vi "FGV.vi"(0 "queue in":refnum<queue>, 1 "Action":enum16{"Get", "Set", "Clear"}(ring), 2 "Logger Name":string, 5 "Logger Output in":T1, 7 "Destroy Logger in":bool=TRUE, 9 "Writer ref in":refnum<vi>, 11 "error in (no error)":errorcluster) -> (4 "queue out":refnum<queue>, 6 "Logger Outputs":T1[](array[typedef]), 8 "Destroy Logger out":bool, 10 "Writer ref out":refnum<vi>, 14 "All Named Loggers":variant, 15 "error out":errorcluster)   [LabVIEW 2016, in "Global_logger.lvlib"]
uses:
  Global_logger.lvlib
  Event.ctl
  Levels.ctl
  Logger Output.ctl
  Level Meaning.ctl
  Sorting.ctl
  Logger Type.ctl
  Log Fields.ctl
  <vilib>/Utility/error.llb/Error Cluster From Error Code.vi
  <vilib>/ErrorRing/Error Ring.xnode
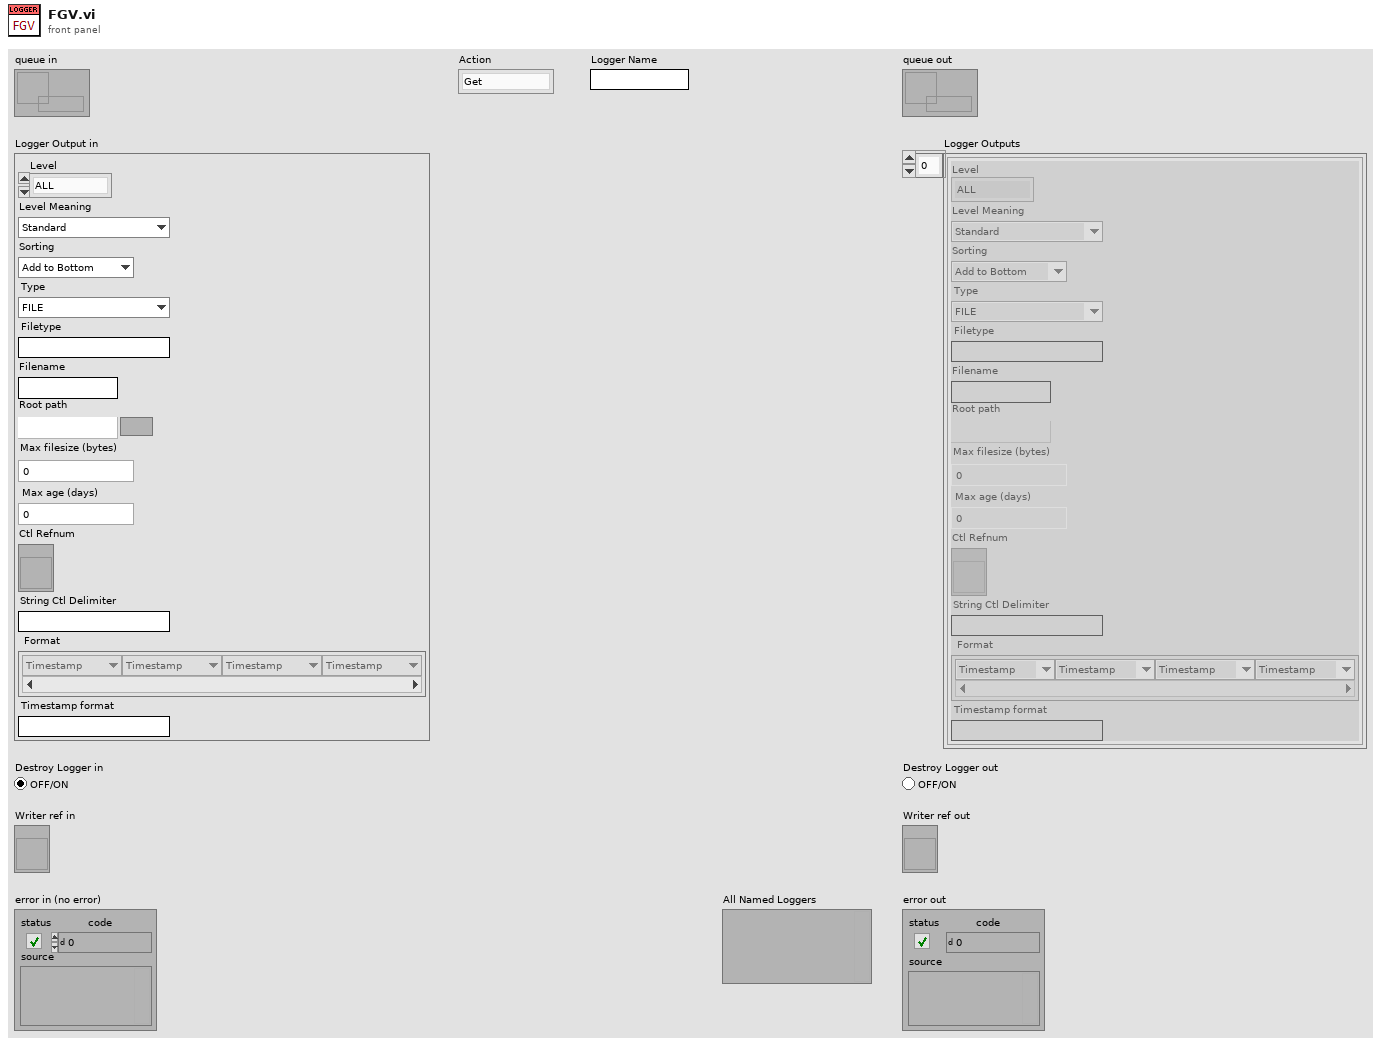
[diagram p1: front panel]
types:
  T1 = typedef "Global_logger.lvlib/Logger Output.ctl" = cluster{"Level":T2, "Level Meaning":T3, "Sorting":T4, "Type":T5, "Filetype":string, "Filename":string, "Root path":path, "Max filesize (bytes)":i32, "Max age (days)":i32, "Ctl Refnum":refnum<vi>, "String Ctl Delimiter":string, "Format":T6[], "Timestamp format":string}
  T2 = typedef "Global_logger.lvlib/Levels.ctl" = enum16{"ALL", "TRACE", "DEBUG", "INFO", "WARN", "ERROR", "FATAL", "OFF"}
  T3 = typedef "Global_logger.lvlib/Level Meaning.ctl" = enum16{"Standard", "Positive", "Exact"}
  T4 = typedef "Global_logger.lvlib/Sorting.ctl" = enum16{"Add to Bottom", "Add to Top"}
  T5 = typedef "Global_logger.lvlib/Logger Type.ctl" = enum16{"FILE", "UI"}
  T6 = typedef "Global_logger.lvlib/Log Fields.ctl" = enum16{"Timestamp", "Level", "Message", "Source VI", "Source App", "Logger Name"}
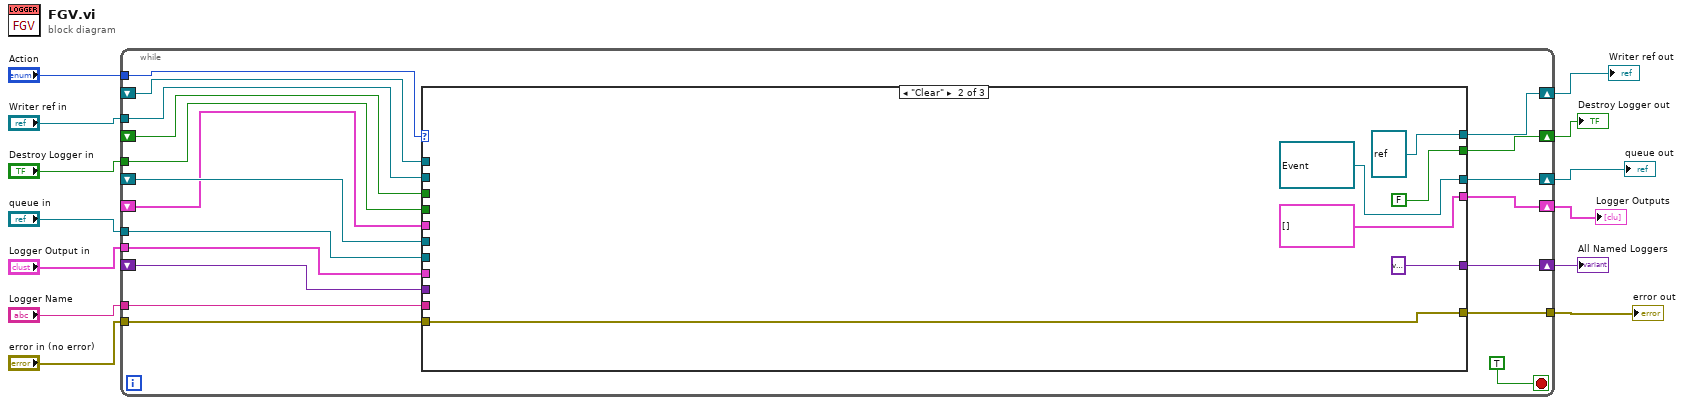
[diagram p0: block diagram]
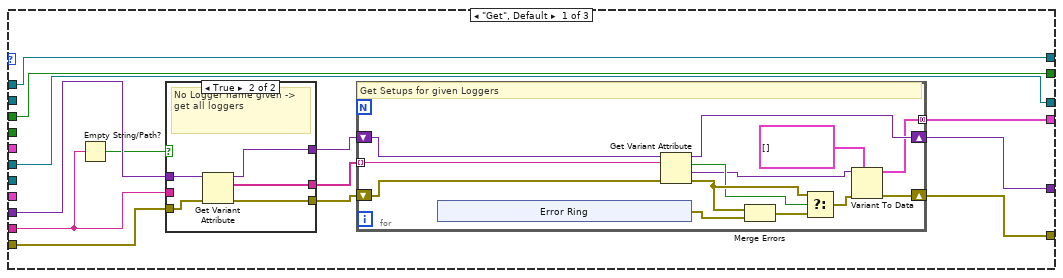
[diagram p2: hidden frame]
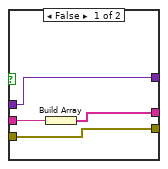
[diagram p3: hidden frame]
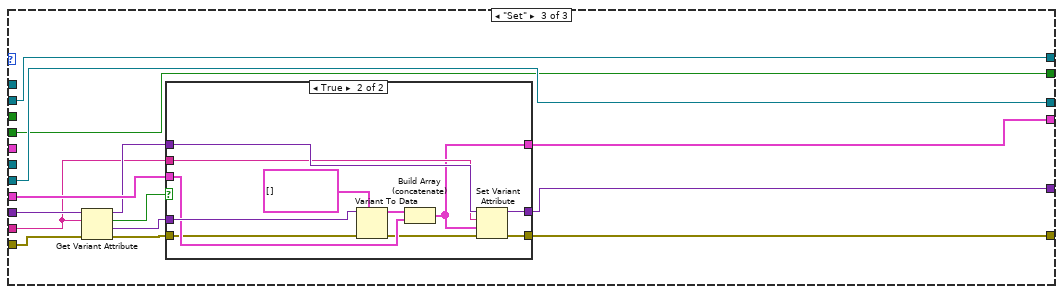
[diagram p4: hidden frame]
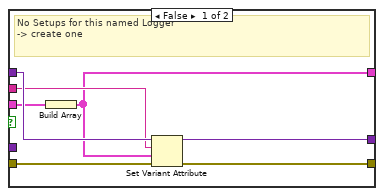
[diagram p5: hidden frame]
diagram:
  n1 = while {
    tunnel: "queue in" -> [w29]
    tunnel: "Action" -> [w31]
    shift-right: [w30] -> w12
    shift-left: _ -> [w28]
    tunnel: "Logger Output in" -> [w26]
    shift-right: [w27] -> w4
    shift-left: _ -> [w25]
    tunnel: "Destroy Logger in" -> [w24]
    shift-right: [w23] -> w10
    shift-left: _ -> [w22]
    shift-right: [w20] -> w3
    shift-left: _ -> [w21]
    tunnel: "Logger Name" -> [w19]
    tunnel: [w18] -> w8
    tunnel: "error in (no error)" -> [w17]
    tunnel: "Writer ref in" -> [w15]
    shift-right: [w16] -> w5
    shift-left: _ -> [w14]
    stop <- TRUE stop-if-true
    n2 = case shown="\"Clear\"" w31 {
      tunnel: [w45 refnum<queue> refnum ("queue in") w91] -> w30
      tunnel: w29 -> [_ _ w91]
      tunnel: w28 -> [w45 _ _]
      tunnel: [w40 T1[] [] w78] -> w27
      tunnel: w26 -> [_ _ w84]
      tunnel: w25 -> [_ _ _]
      tunnel: w24 -> [_ _ w90]
      tunnel: [w44 FALSE ("Destroy Logger in") w90] -> w23
      tunnel: w22 -> [w44 _ _]
      tunnel: w21 -> [w39 _ w89]
      tunnel: [w42 variant w79] -> w20
      tunnel: w19 -> [w34 _ w81]
      tunnel: [w41 w77 w80] -> w18
      tunnel: w17 -> [w37 w77 w88]
      tunnel: [w43 refnum<vi> refnum ("Writer ref in") w87] -> w16
      tunnel: w15 -> [_ _ w87]
      tunnel: w14 -> [w43 _ _]
      frame "Get", Default {
        n3 = Empty String/Path?(string/path=w34) -> (empty?=w35:bool)
        n4 = case shown="True" w35 {
          tunnel: w39 -> [w65 w71]
          tunnel: [w65 w70] -> w38
          tunnel: w37 -> [w66 w69]
          tunnel: [w66 w68] -> w36
          tunnel: w34 -> [w64 _]
          tunnel: [w63 w67] -> w33
          frame False {
            n5 = Build Array(w64) -> (w63:string[])
          }
          frame True {
            # "No Logger name given -> get all loggers"
            n6 = Get Variant Attribute(Variant=w71, error in=w69) -> (duplicate Variant=w70:variant, names=w67:string[], error out=w68:errorcluster)  [unwired: 2 in, 1 out]
          }
        }
        n7 = for {
          tunnel: [w49] -> w40 mode=concatenating
          tunnel: w33 -> [w48] mode=indexing
          shift-right: [w58] -> w42
          shift-left: w38 -> [w47]
          shift-right: [w52] -> w41
          shift-left: w36 -> [w46]
          # "Get Setups for given Loggers"
          n8 = xnode "Error Ring"() -> ("error out"=w57:errorcluster)
          n9 = Get Variant Attribute(Variant=w47, name=w48, error in=w46) -> (duplicate Variant=w58:variant, found=w54:bool, value=w51:variant, error out=w55:errorcluster)  [unwired: 1 in]
          n10 = Merge Errors(w55, w57) -> (w56:errorcluster)
          n11 = Select(t=w55, s=w54, f=w56) -> (s? t:f=w53:errorcluster)
          n12 = Variant To Data(error in=w53, type=T1[] [], Variant=w51) -> (data=w49:T1[], error out=w52:errorcluster)
        }
      }
      frame "Clear" {
      }
      frame "Set" {
        n13 = Get Variant Attribute(Variant=w89, name=w81, error in=w88) -> (duplicate Variant=w82:variant, found=w86:bool, value=w85:variant, error out=w83:errorcluster)  [unwired: 1 in]
        n14 = case shown="True" w86 {
          tunnel: w85 -> [_ w109]
          tunnel: w84 -> [w94 w107]
          tunnel: w83 -> [w98 w106]
          tunnel: w82 -> [w96 w104]
          tunnel: w81 -> [w93 w103]
          tunnel: [w97 w102] -> w80
          tunnel: [w95 w101] -> w79
          tunnel: [w92 w100] -> w78
          frame False {
            # "No Setups for this named Logger\n-> create one"
            n15 = Build Array(w94) -> (w92:T1[])
            n16 = Set Variant Attribute(Variant=w96, name=w93, value=w92, error in=w98) -> (Variant out=w95:variant, error out=w97:errorcluster)  [unwired: 1 out]
          }
          frame True {
            n17 = Variant To Data(error in=w106, type=T1[] [], Variant=w109) -> (data=w108:T1[], error out=w105:errorcluster)
            n18 = Build Array (concatenate)(w108, w107) -> (w100:T1[])
            n19 = Set Variant Attribute(Variant=w104, name=w103, value=w100, error in=w105) -> (Variant out=w101:variant, error out=w102:errorcluster)  [unwired: 1 out]
          }
        }
      }
    }
  }
  "queue out" <- w12
  "error out" <- w8
  "Destroy Logger out" <- w10
  "Writer ref out" <- w5
  "Logger Outputs" <- w4
  "All Named Loggers" <- w3
